vi "BlinkM GetAddress.vi"(8 "Error In":errorcluster, 10 "Address (0)":u8, 11 "ChipKit Resource":T1={"COM Port"="", "Board Type"=enum."ChipKit uC32", "Connection Type"=enum."USB / Serial", "Baud Rate (115200)"=15, "Bytes Per Packet (15)"=15}) -> (0 "Error Out":errorcluster, 2 "BlinkM Address":u8, 3 "ChipKit Resource":T1={"COM Port"="", "Board Type"=enum."ChipKit uC32", "Connection Type"=enum."USB / Serial", "Baud Rate (115200)"=15, "Bytes Per Packet (15)"=15})   [LabVIEW 2011, in "LabVIEW Interface for ChipKit.lvlib"]
doc: "Get the address of the BlinkM. This VI can be used to determine the address of a single BlinkM on the I2C bus using the general call address (0x00)."
uses:
  LabVIEW Interface for ChipKit.lvlib
  Private/Type Defs/Board Type.ctl
  Private/Type Defs/Chipkit Resource.ctl
  Private/Type Defs/Connection Type.ctl
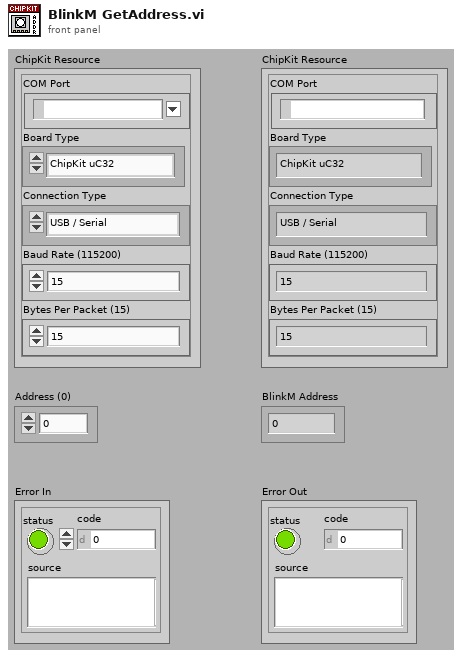
[diagram p1: front panel]
types:
  T1 = typedef "LabVIEW Interface for ChipKit.lvlib/Chipkit Resource.ctl" = cluster{"COM Port":refnum<visa-resource-name>, "Board Type":T2, "Connection Type":T3, "Baud Rate (115200)":u32, "Bytes Per Packet (15)":u32}
  T2 = typedef "LabVIEW Interface for ChipKit.lvlib/Board Type.ctl" = enum16{"ChipKit uC32", "ChipKit Uno32", "ChipKit Max32"}
  T3 = typedef "LabVIEW Interface for ChipKit.lvlib/Connection Type.ctl" = enum8{"USB / Serial", "XBEE", "BlueSmirf (Bluetooth)"}
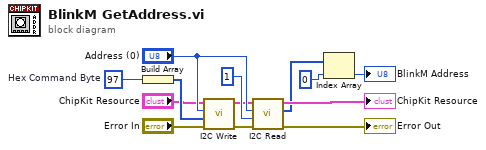
[diagram p0: block diagram]
diagram:
  w12 = u8 97  # Hex Command Byte
  n1 = Build Array(w12) -> (w11:u8[])
  n2 = call "I2C Write.vi"("Error In"="Error In", "I2C Data"=w11, "Address (0)"="Address (0)", "ChipKit Resource"="ChipKit Resource") -> ("Error Out"=w10:errorcluster, "ChipKit Resource"=w5:T1)  [unwired: 6 in]
  n3 = call "I2C Read.vi"("Error In"=w10, "Bytes To Read"=u8 1, "Address (0)"="Address (0)", "ChipKit Resource"=w5) -> ("Error Out"=→"Error Out":errorcluster, "I2C Data"=w1:u8[], "ChipKit Resource"=→"ChipKit Resource":T1)  [unwired: 5 in]
  n4 = Index Array(array=w1, index=0) -> (element=→"BlinkM Address":u8)
